vi "Open Dynamic VI References.vi"(8 "error in (no error)":errorcluster, 11 "Tx Scheduled Labels Execution Unit in":refnum<class "Tx Scheduled Labels Execution Unit.lvclass">) -> (0 "error out":errorcluster, 3 "Tx Scheduled Labels Execution Unit out":refnum<class "Tx Scheduled Labels Execution Unit.lvclass">)   [LabVIEW 2020, in "Ballard ARINC 429 Engine.lvlib" / "Implementation.lvlib" / "Tx Scheduled Labels Execution Unit.lvclass"]
uses:
  Tx Scheduled Labels Execution Unit.lvclass
  Tx Scheduled Labels Execution Unit.lvclass/Tx Scheduled Labels Execution Unit.ctl
  Check Previous Values.vi
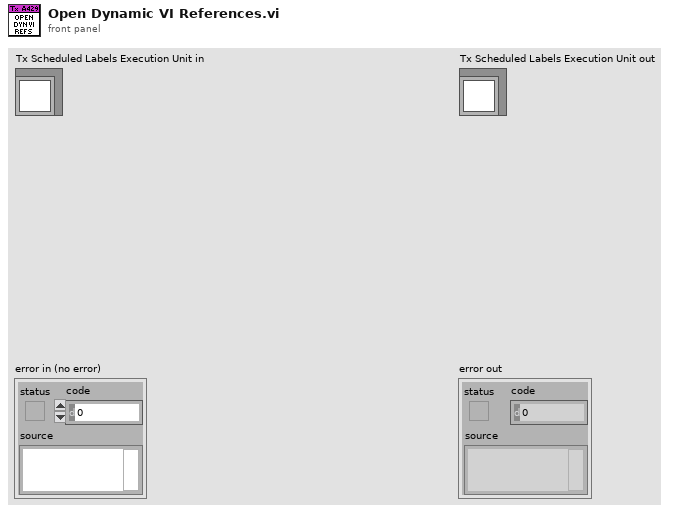
[diagram p1: front panel]
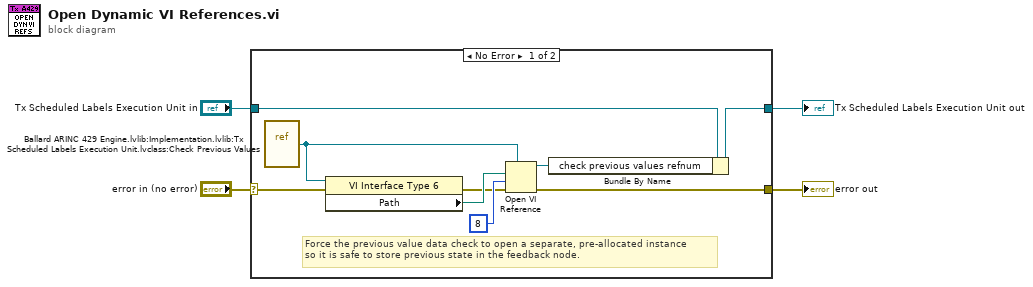
[diagram p0: block diagram]
diagram:
  n1 = case shown="No Error" "error in (no error)" {
    selector: "error in (no error)" -> [w9 w15]
    tunnel: [w5 w15] -> w3
    tunnel: [w10 w14] -> w1
    tunnel: "Tx Scheduled Labels Execution Unit in" -> [w11 w14]
    frame No Error {
      # "Force the previous value data check to open a separate, pre-allocated instance\nso it is safe to store previous state in the feedback node."
      n2 = vi-ref "Ballard ARINC 429 Engine.lvlib:Implementation.lvlib:Tx Scheduled Labels Execution Unit.lvclass:Check Previous Values.vi"() -> (w7:refnum<vi>)
      n3 = property class="VI Interface Type 6"(reference=w7, error in=w9) -> (error out=w8:errorcluster, "Path"=w12:path)  [unwired: 1 out]
      n4 = Open VI Reference(type specifier VI Refnum (for type only)=w7, vi path=w12, options=8, error in (no error)=w8) -> (vi reference=w6:refnum<vi>, error out=w5:errorcluster)  [unwired: 2 in]
      n5 = Bundle By Name(cluster=w11, "check previous values refnum"=w6) -> (w10:refnum<class "Tx Scheduled Labels Execution Unit.lvclass">)
    }
    frame Error {
    }
  }
  "error out" <- w3
  "Tx Scheduled Labels Execution Unit out" <- w1
